vi "Enigma plugboard.vi"(1 "Pistoketaulu":string[][](array[string]), 2 "Merkki sisään":string) -> (0 "Merkki ulos":string)   [LabVIEW 2023]
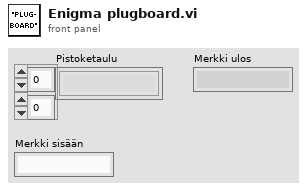
[diagram p1: front panel]
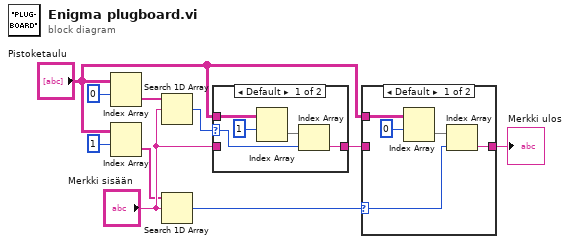
[diagram p0: block diagram]
diagram:
  n1 = Index Array(array="Pistoketaulu", index (row)=0) -> (element=w5:string[])  [unwired: 1 in]
  n2 = Index Array(array="Pistoketaulu", index (row)=1) -> (element=w1:string[])  [unwired: 1 in]
  n3 = Search 1D Array(1D array=w5, element="Merkki sisään") -> (index of element=w6:i32)  [unwired: 1 in]
  n4 = Search 1D Array(1D array=w1, element="Merkki sisään") -> (index of element=w2:i32)  [unwired: 1 in]
  n5 = case "Plugboard" shown="Default" w6 {
    selector: w6 -> [w13 _]
    tunnel: "Merkki sisään" -> [_ w16]
    tunnel: [w12 w16] -> w8
    tunnel: "Pistoketaulu" -> [w15 _]
    frame Default {
      n6 = Index Array(array=w15, index (row)=1 ("index (col)")) -> (element=w14:string[])  [unwired: 1 in]
      n7 = Index Array(array=w14, index=w13) -> (element=w12:string)
    }
    frame -1 {
    }
  }
  n8 = case "Plugboard" shown="Default" w2 {
    selector: w2 -> [w19 _]
    tunnel: w8 -> [_ w22]
    tunnel: [w18 w22] -> w3
    tunnel: "Pistoketaulu" -> [w21 _]
    frame Default {
      n9 = Index Array(array=w21, index (row)=0 ("index (col)")) -> (element=w20:string[])  [unwired: 1 in]
      n10 = Index Array(array=w20, index=w19) -> (element=w18:string)
    }
    frame -1 {
    }
  }
  "Merkki ulos" <- w3
